vi "AudioAnalyzer_with_AnalogDiscovery2.vi"() -> ()   [LabVIEW 2020]
uses:
  <vilib>/express/express analysis/Spectral/Block/exnSpectralBlock spectral measurements RMS poly.vi
  <vilib>/express/express analysis/Spectral/Block/exnSpectralBlock spectral measurements RMS array WFM.vi
  <vilib>/express/express analysis/Spectral/XNode/ExpressSpectralMeasurementsBlockNode.xnode
  <vilib>/DigilentWF/DigilentWF.lvlib
panel:
  out "P-P [V]":dbl format="%.6g"
  out "Frequency [Hz]":dbl format="%#.4f"
  out "Spectrum":cluster{"f0":dbl, "df":dbl, "magnitude":dbl[]}[](graph)
  out "Waveform Graph":waveform(dbl)[](graph)
  out "RMS [V]":dbl
  out "SINAD [dB]":dbl format="%#.2f"
  out "SINAD [dB]":dbl(knob) scale=0.0..24.0
  in  "Range [V]":string(combo)
  out "Distortion [%]":dbl format="%#_4f"
  out "Status":i32(ring) items=["Stopped", "Running", "Triggered", "Acquisition Complete"]
  out "Trigger Reason":i32(ring) items=["Normal", "Forced", "Auto"]
  out "Error Out":errorcluster
  in  "stop":bool
  # "Audio Analyzer with AnalogDiscovery2"
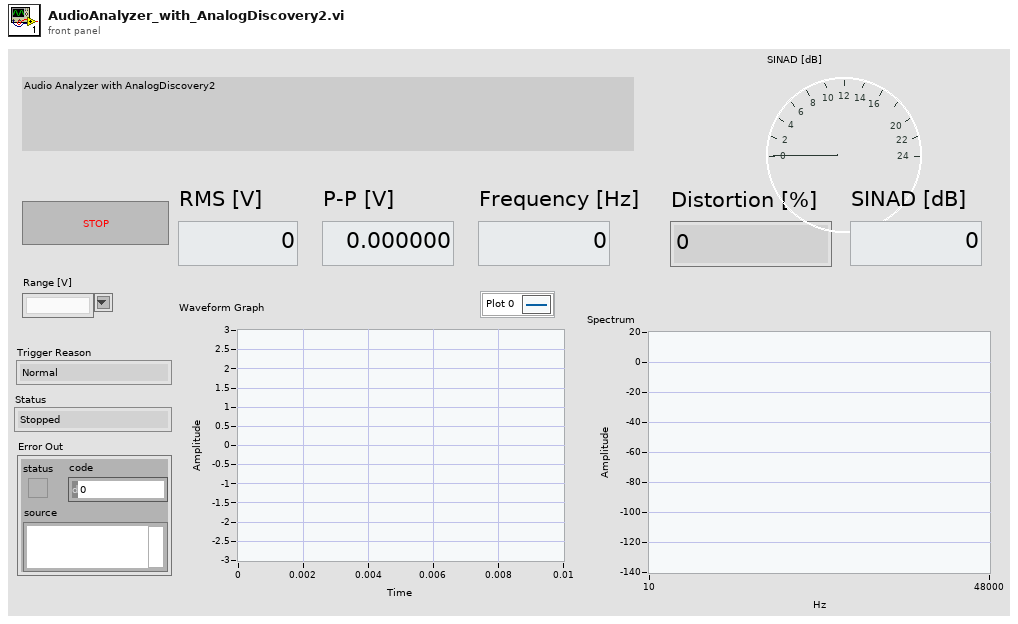
[diagram p1: front panel]
types:
  T1 = cluster{"averaging mode":u16, "weighting mode":u16, "number of averages":u32}
  T2 = cluster{"dB On (F)":bool, "unwrap phase (F)":bool, "convert to degree (F)":bool}
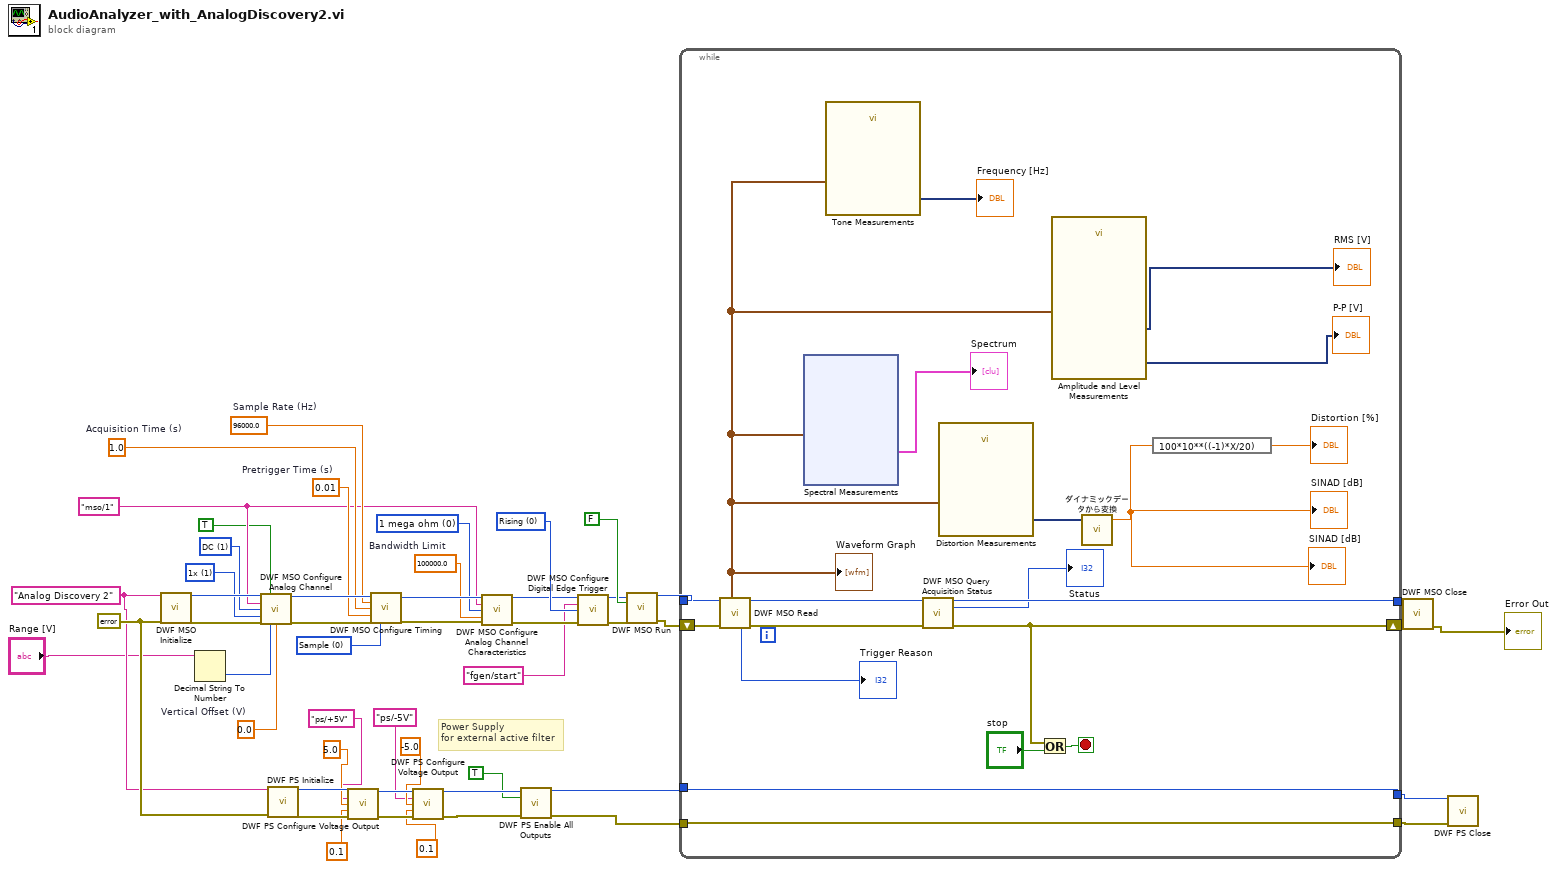
[diagram p0: block diagram]
diagram:
  w47 = 0.0  # Vertical Offset (V)
  w44 = 1.0  # Acquisition Time (s)
  w45 = 96000.0  # Sample Rate (Hz)
  w21 = errorcluster {"status"=FALSE, "code"=0, "source"=""} ("Error In")
  w35 = 0 items=["Sample", "Peak Detect"] ("Sampling Mode")
  w36 = 0 items=["Rising", "Falling", "Either"] ("Trigger Slope")
  w38 = 100000.0  # Bandwidth Limit
  w39 = 0 items=["1 mega ohm", "50 ohms"] ("Input Impedance")
  w42 = 0.01  # Pretrigger Time (s)
  w48 = 1 items=["1x"=1, "10x"=10] ("Probe Attenuation")
  w49 = 1 items=["AC", "DC"] ("Vertical Coupling")
  w40 = "mso/1" ("Channel")
  w3 = "Analog Discovery 2" ("Device Name")
  # "Power Supply\nfor external active filter"
  n1 = call <vilib>:"DWF MSO Initialize.vi"("Device Name"=w3, "Error In"=w21) -> ("Instrument Handle Out"=w50:u32, "Error Out"=w32:errorcluster)  [unwired: 12 in]
  n2 = Decimal String To Number(string="Range [V]") -> (number=w1:i32)  [unwired: 2 in, 1 out]
  n3 = call <vilib>:"DWF MSO Configure Analog Channel.vi"("Instrument Handle In"=w50, "Enable Channel"=TRUE, "Channel"=w40, "Vertical Coupling"=w49, "Probe Attenuation"=w48, "Error In"=w32, "Vertical Range"=w1, "Vertical Offset"=w47) -> ("Instrument Handle Out"=w46:u32, "Error Out"=w43:errorcluster)  [unwired: 6 in]
  n4 = call <vilib>:"DWF PS Initialize.vi"("Device Name"=w3, "Error In"=w21) -> ("Instrument Handle Out"=w12:u32, "Error Out"=w13:errorcluster)  [unwired: 12 in]
  n5 = call <vilib>:"DWF PS Configure Voltage Output.vi"("Instrument Handle In"=w12, "Channel"="ps/+5V" ("Trigger Source"), "Voltage Level"=5.0, "Current Limit"=0.1, "Error In"=w13) -> ("Instrument Handle Out"=w11:u32, "Error Out"=w14:errorcluster)  [unwired: 9 in]
  n6 = call <vilib>:"DWF MSO Configure Timing.vi"("Instrument Handle In"=w46, "Sample Rate"=w45, "Acquisition Time (s)"=w44, "Pretrigger Time (s)"=w42, "Error In"=w43, "Sampling Mode"=w35) -> ("Instrument Handle Out"=w41:u32, "Error Out"=w37:errorcluster)  [unwired: 8 in]
  n7 = call <vilib>:"DWF PS Configure Voltage Output.vi"("Instrument Handle In"=w11, "Channel"="ps/-5V" ("Trigger Source"), "Voltage Level"=-5.0, "Current Limit"=0.1, "Error In"=w14) -> ("Instrument Handle Out"=w19:u32, "Error Out"=w15:errorcluster)  [unwired: 9 in]
  n8 = call <vilib>:"DWF MSO Configure Analog Channel Characteristics.vi"("Instrument Handle In"=w41, "Channel"=w40, "Input Impedance"=w39, "Bandwidth Limit"=w38, "Error In"=w37) -> ("Instrument Handle Out"=w30:u32, "Error Out"=w31:errorcluster)  [unwired: 9 in]
  n9 = call <vilib>:"DWF PS Enable All Outputs.vi"("Instrument Handle In"=w19, "Enable Outputs"=TRUE, "Error In"=w15) -> ("Instrument Handle Out"=w18:u32, "Error Out"=w20:errorcluster)  [unwired: 11 in]
  n10 = call <vilib>:"DWF MSO Configure Digital Edge Trigger.vi"("Instrument Handle In"=w30, "Trigger Source"="fgen/start", "Trigger Slope"=w36, "Error In"=w31) -> ("Instrument Handle Out"=w26:u32, "Error Out"=w24:errorcluster)  [unwired: 10 in]
  n11 = call <vilib>:"DWF MSO Run.vi"("Instrument Handle In"=w26, "Auto Trigger"=FALSE, "Error In"=w24) -> ("Instrument Handle Out"=w28:u32, "Error Out"=w23:errorcluster)  [unwired: 11 in]
  n12 = while {
    tunnel: w28 -> [w65]
    tunnel: [w66] -> w33
    shift-right: [w63] -> w29
    shift-left: w23 -> [w62]
    tunnel: w20 -> [w58]
    tunnel: w18 -> [w51]
    tunnel: [w58] -> w17
    tunnel: [w51] -> w16
    stop <- w61 stop-if-true
    n13 = call <vilib>:"DWF MSO Read.vi"("Instrument Handle In"=w65, "Error In"=w62) -> ("Instrument Handle Out"=w67:u32, "Analog Waveforms"=w53:waveform(dbl)[], "Trigger Reason"=→"Trigger Reason":i32, "Error Out"=w68:errorcluster)  [unwired: 8 in, 2 out]
    "Waveform Graph" <- w53
    n14 = xnode "Spectral Measurements"("Signals"=w53) -> ("FFT - (RMS)"=→"Spectrum":cluster{"f0":dbl, "df":dbl, "magnitude":dbl[]}[])  [unwired: 1 in, 2 out]
    n15 = call "Tone Measurements"("Signals"=w53) -> ("Frequency"=→"Frequency [Hz]":dynamicdata)  [unwired: 9 in, 1 out]
    n16 = call <vilib>:"DWF MSO Query Acquisition Status.vi"("Instrument Handle In"=w67, "Error In"=w68) -> ("Instrument Handle Out"=w66:u32, "Status"=→"Status":i32, "Error Out"=w63:errorcluster)  [unwired: 11 in]
    n17 = call "Distortion Measurements"("Signals"=w53) -> ("SINAD (dB)"=w59:dynamicdata)  [unwired: 9 in, 1 out]
    n18 = Or(x=w63, y="stop") -> (x .or. y?=w61:bool)
    n19 = call "Amplitude and Level Measurements"("Signals"=w53) -> ("RMS"=→"RMS [V]":dynamicdata, "Peak to Peak"=→"P-P [V]":dynamicdata)  [unwired: 11 in, 2 out]
    n20 = call "ダイナミックデータから変換"("Dynamic Data Type"=w59) -> ("Scalar"=w57:dbl)  [unwired: 1 in, 2 out]
    "SINAD [dB]" <- w57
    "SINAD [dB]" <- w57
    n21 = expression code="100*10**((-1)*X/20)"(w57) -> (→"Distortion [%]":dbl)
  }
  n22 = call <vilib>:"DWF MSO Close.vi"("Instrument Handle In"=w33, "Error In"=w29) -> ("Error Out"=→"Error Out":errorcluster)  [unwired: 13 in]
  n23 = call <vilib>:"DWF PS Close.vi"("Instrument Handle In"=w16, "Error In"=w17) -> ()  [unwired: 13 in, 1 out]
